vi "Remove Children.vi"(8 "error in (no error)":errorcluster, 11 "Config Element in":refnum<class "Config Element.lvclass">) -> (0 "error out":errorcluster, 3 "Config Element out":refnum<class "Config Element.lvclass">)   [LabVIEW 2023, in "CDM-Config.lvlib" / "Config Element.lvclass"]
uses:
  Config Element.lvclass
  Config Element.lvclass/Config Element.ctl
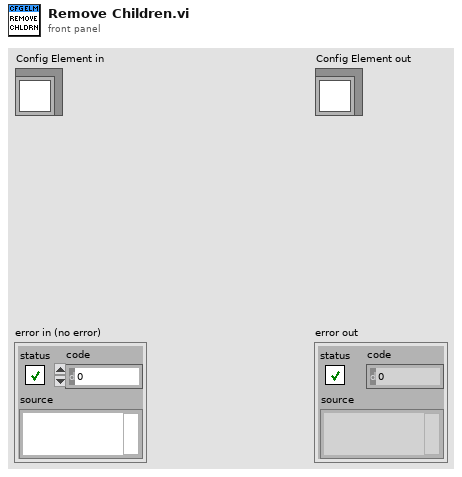
[diagram p1: front panel]
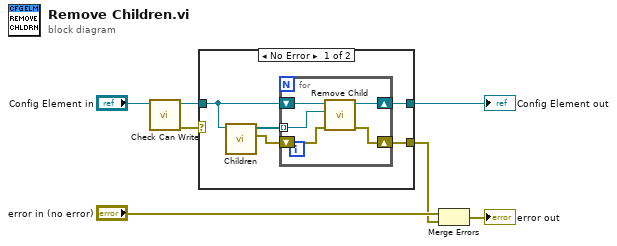
[diagram p0: block diagram]
diagram:
  n1 = call "Check Can Write.vi"("Config Element in"="Config Element in") -> ("error out"=w1:errorcluster, "Config Element out"=w2:refnum<class "Config Element.lvclass">)  [unwired: 9 in]
  n2 = case shown="No Error" w1 {
    selector: w1 -> [_ w18]
    tunnel: [w10 w19] -> w5
    tunnel: [w9 w18] -> w3
    tunnel: w2 -> [w8 w19]
    frame No Error {
      n3 = call "Children.vi"("Config Element in"=w8) -> ("error out"=w11:errorcluster, "Elements"=w12:refnum<class "Config Element.lvclass">[])  [unwired: 9 in]
      n4 = for {
        tunnel: w12 -> [w16] mode=indexing
        shift-right: [w14] -> w9
        shift-left: w11 -> [w15]
        shift-right: [w13] -> w10
        shift-left: w8 -> [w17]
        n5 = call "Remove Child.vi"("error in (no error)"=w15, "Child"=w16, "Config Element in"=w17) -> ("error out"=w14:errorcluster, "Config Element out"=w13:refnum<class "Config Element.lvclass">)  [unwired: 7 in]
      }
    }
    frame Error {
    }
  }
  "Config Element out" <- w5
  n6 = Merge Errors("error in (no error)", w3) -> (→"error out":errorcluster)
